vi "m1m3_logEvent_ILCWarning.vi"(8 "error in (no error)":errorcluster, 11 "logevent_ILCWarning_Ctl":T1) -> (0 "error out":errorcluster, 2 "function return":i32, 3 "logevent_ILCWarning_Ctl out":T1)   [LabVIEW 2016, in "SALLV_m1m3.lvlib"]
doc: "int m1m3_shm_logEvent_ILCWarningLV(m1m3_logevent_ILCWarningLV *logevent_ILCWarning_Ctl );"
uses:
  SALLV_m1m3.lvlib
  DataTypes/logevent_ILCWarning.ctl
  SALLV_m1m3.so
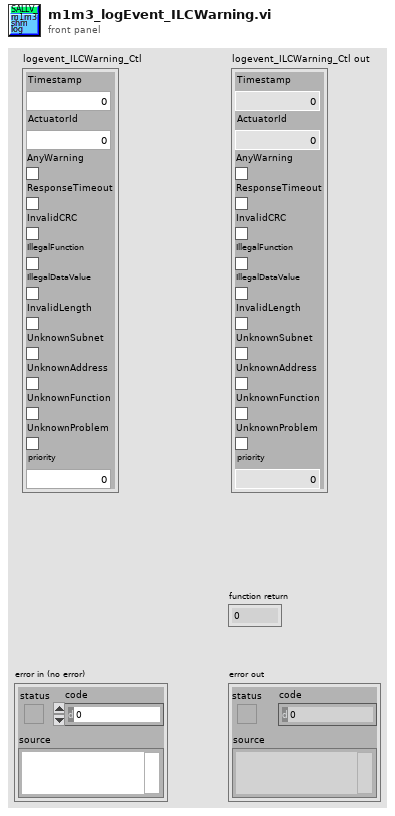
[diagram p1: front panel]
types:
  T1 = typedef "SALLV_m1m3.lvlib/logevent_ILCWarning.ctl" = cluster{"Timestamp":dbl, "ActuatorId":i32, "AnyWarning":bool, "ResponseTimeout":bool, "InvalidCRC":bool, "IllegalFunction":bool, "IllegalDataValue":bool, "InvalidLength":bool, "UnknownSubnet":bool, "UnknownAddress":bool, "UnknownFunction":bool, "UnknownProblem":bool, "priority":i32}
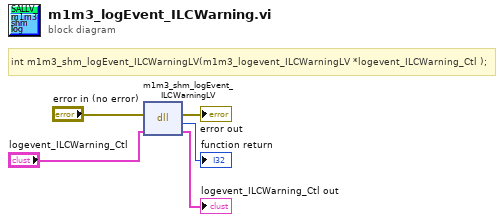
[diagram p0: block diagram]
diagram:
  # "int m1m3_shm_logEvent_ILCWarningLV(m1m3_logevent_ILCWarningLV *logevent_ILCWarning_Ctl );"
  n1 = dll-call lib="opt/CODE/SALLV_m1m3/SALLV_m1m3.*" fn="m1m3_shm_logEvent_ILCWarningLV"(error in="error in (no error)", "logevent_ILCWarning_Ctl"="logevent_ILCWarning_Ctl") -> (error out=→"error out":errorcluster, →"function return":i32, "logevent_ILCWarning_Ctl"=→"logevent_ILCWarning_Ctl out":T1)  [unwired: 2 in, 1 out]
